vi "Select Role Prompt.vi"(10 "Available Roles":string[](array[string])) -> (1 "Selected Role":string, 2 "Cancelled":bool)   [LabVIEW 2020, in "VolatusGUI.lvlib" / "GUI Manager Module.lvclass"]
uses:
  GUI Manager Module.lvclass
  GUI Manager Module.lvclass/GUI Manager Module.ctl
panel:
  in  "Cancel":bool
  in  "Accept":bool
  in  "Roles":i32(listbox)
  # "Select role to login as:"
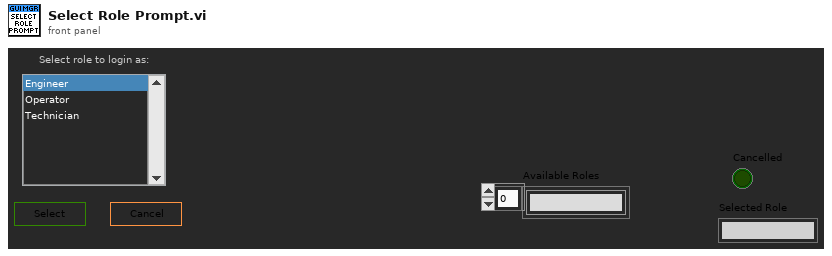
[diagram p1: front panel]
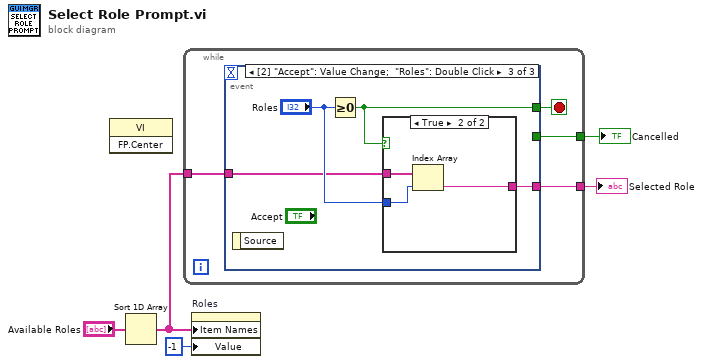
[diagram p0: block diagram]
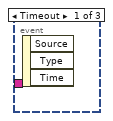
[diagram p2: hidden frame]
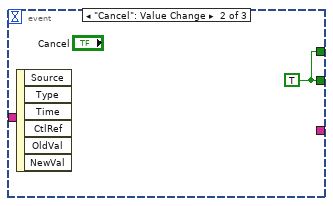
[diagram p3: hidden frame]
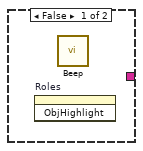
[diagram p4: hidden frame]
diagram:
  n1 = invoke class="VI" method="FP.Center"() -> ()  [unwired: 3 in, 3 out]
  n2 = Sort 1D Array(array="Available Roles") -> (sorted array=w2:string[])
  n3 = while {
    tunnel: [w9] -> w3
    tunnel: w2 -> [w7]
    tunnel: [w6] -> w1
    stop <- w8 stop-if-true
    n4 = event shown="[2] \"Accept\": Value Change;  \"Roles\": Double Click" {
      selector: _ -> [_ _ _]
      dyn-events: _ -> [_ _ _]
      timeout: _ -> [_ _ _]
      tunnel: [_ w10 _] -> w9
      tunnel: [_ w10 w14] -> w8
      tunnel: w7 -> [_ _ w12]
      tunnel: [_ _ w11] -> w6
      event Timeout {
        n5 = event-data() -> ()  [unwired: 1 in, 3 out]
      }
      event "Cancel": Value Change {
        w10 = TRUE
        n6 = event-data() -> ()  [unwired: 1 in, 6 out]
      }
      event "Accept": Value Change; "Roles": Double Click {
        n7 = event-data() -> ()  [unwired: 1 in, 1 out]
        n8 = Greater Or Equal To 0?(x="Roles") -> (x >= 0?=w14:bool)
        n9 = case shown="True" w14 {
          tunnel: "Roles" -> [_ w16]
          tunnel: w12 -> [_ w17]
          tunnel: [_ w15] -> w11
          frame False {
            n10 = invoke on="Roles" class="LstBox (strict)" method="ObjHighlight"() -> ()  [unwired: 3 in, 3 out]
            n11 = call <vilib>:"Beep.vi"() -> ()  [unwired: 12 in]
          }
          frame True {
            n12 = Index Array(array=w17, index=w16) -> (element=w15:string)
          }
        }
      }
    }
  }
  "Cancelled" <- w3
  "Selected Role" <- w1
  n13 = property on="Roles" class="LstBox (strict)"("Item Names"=w2, "Value"=-1 ("Roles")) -> ()  [unwired: 2 in, 2 out]
